vi "Load Log.vi"(11 "selected path":path) -> (2 "Log Data":cluster{refnum<class "RDS State.lvclass">[]}[](array[cluster]), 3 "Log Header":T1, 5 "size(s)":i32)   [LabVIEW 2015, in "Log Waveform Processors.lvlib"]
uses:
  Log Waveform Processors.lvlib
  Actors/RDS Logger Actor/RDS Logger Actor/RDS Logger Actor/Logger Header.ctl
  RDS State Tracker/RDS State/RDS State.lvclass
panel:
  # "Opening Log..."
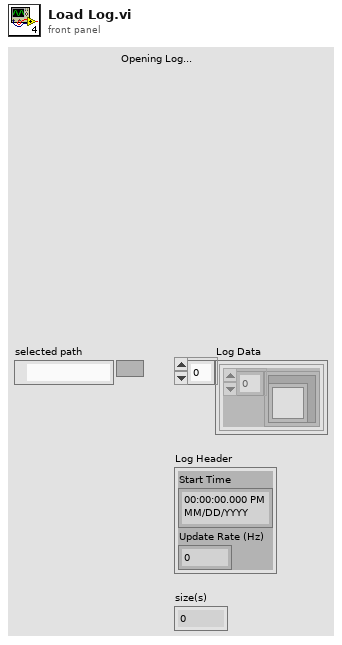
[diagram p1: front panel]
types:
  T1 = typedef "Log Waveform Processors.lvlib/Logger Header.ctl" = cluster{"Start Time":timestamp, "Update Rate (Hz)":dbl}
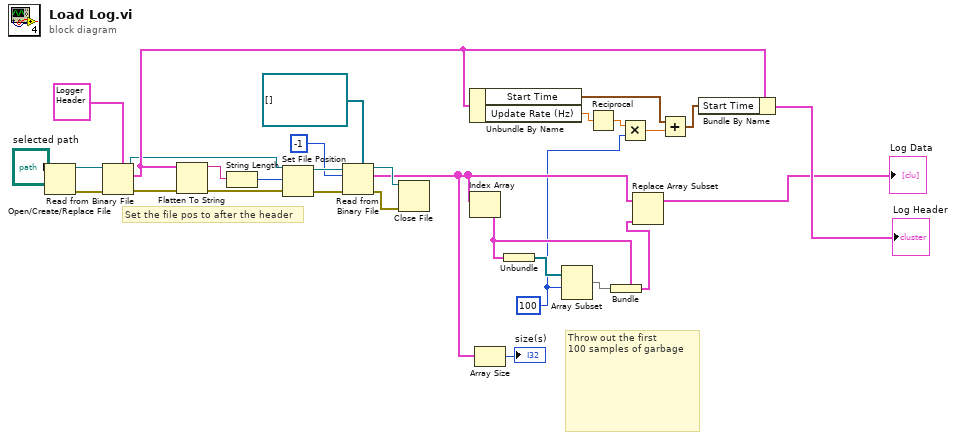
[diagram p0: block diagram]
diagram:
  w17 = 100 ("index")
  # "Throw out the first \n100 samples of garbage"
  # "Set the file pos to after the header"
  n1 = Open/Create/Replace File(file path (use dialog)="selected path") -> (refnum out=w7:refnum<file>, error out=w6:errorcluster)  [unwired: 5 in, 1 out]
  n2 = Read from Binary File(5:T1 {"Start Time"=timestamp(0 s since 1904-01-01), "Update Rate (Hz)"=0.0} ("Log Header"), 8:w6, 11:w7) -> (0:w12:errorcluster, 2:w20:T1, 3:w11:refnum<file>)  [unwired: 3 in, 1 out]
  n3 = Flatten To String(anything=w20, error in (no error)=w12) -> (data string=w9:string, error out=w8:errorcluster)  [unwired: 2 in, 1 out]
  n4 = String Length(string=w9) -> (length=w10:i32)
  n5 = Set File Position(offset (in bytes) (0)=w10, refnum=w11, error in=w8) -> (refnum out=w13:refnum<file>, error out=w14:errorcluster)  [unwired: 1 in]
  n6 = Read from Binary File(5:refnum<class "RDS State.lvclass">[] [], 8:w14, 10:-1 ("count (1)"), 11:w13) -> (0:w28:errorcluster, 2:w22:cluster{refnum<class "RDS State.lvclass">[]}[], 3:w27:refnum<file>)  [unwired: 2 in, 1 out]
  n7 = Close File(refnum=w27, error in=w28) -> ()  [unwired: 2 out]
  n8 = Unbundle By Name(w20) -> ("Start Time"=w19:timestamp, "Update Rate (Hz)"=w15:dbl)
  n9 = Index Array(array=w22) -> (element=w24:cluster{refnum<class "RDS State.lvclass">[]})  [unwired: 1 in]
  n10 = Array Size(array=w22) -> (size(s)=→"size(s)":i32)
  n11 = Unbundle(w24) -> (w23:refnum<class "RDS State.lvclass">[])
  n12 = Array Subset(array=w23, index=w17) -> (w25:refnum<class "RDS State.lvclass">[])  [unwired: 1 in]
  n13 = Reciprocal(x=w15) -> (1/x=w16:dbl)
  n14 = Bundle(cluster=w24, w25) -> (w26:cluster{refnum<class "RDS State.lvclass">[]})
  n15 = Multiply(x=w16, y=w17) -> (x*y=w18:dbl)
  n16 = Replace Array Subset(array=w22, new element=w26) -> (→"Log Data":cluster{refnum<class "RDS State.lvclass">[]}[])  [unwired: 1 in]
  n17 = Add(x=w19, y=w18) -> (x+y=w21:timestamp)
  n18 = Bundle By Name(cluster=w20, "Start Time"=w21) -> (→"Log Header":T1)
